vi "InitDrv_thread.vi"() -> (0 "Boards":u8)   [LabVIEW 2015]
uses:
  lv64_eventdriven/board.vis/ESLSCDLL.dll
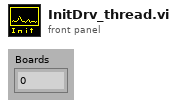
[diagram p1: front panel]
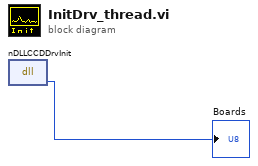
[diagram p0: block diagram]
diagram:
  n1 = dll-call lib="C:/ENTW/PCIE/64bit/lv64/lv64_eventdriven/board.vis/ESLSCDLL.dll" fn="nDLLCCDDrvInit" ("lwlscdll.dll:DLLCCDDrvInit")() -> ("Rückgabetyp"=→"Boards":u8)  [unwired: 3 in, 2 out]
